vi "start.vi"(8 "error in (no error)":errorcluster, 11 "CQT_DDS in":refnum<class "CQT_DDS.lvclass">) -> (0 "error out":errorcluster, 3 "CQT_DDS out":refnum<class "CQT_DDS.lvclass">)   [LabVIEW 2011, in "CQT_DDS.lvclass"]
uses:
  CQT_DDS.lvclass
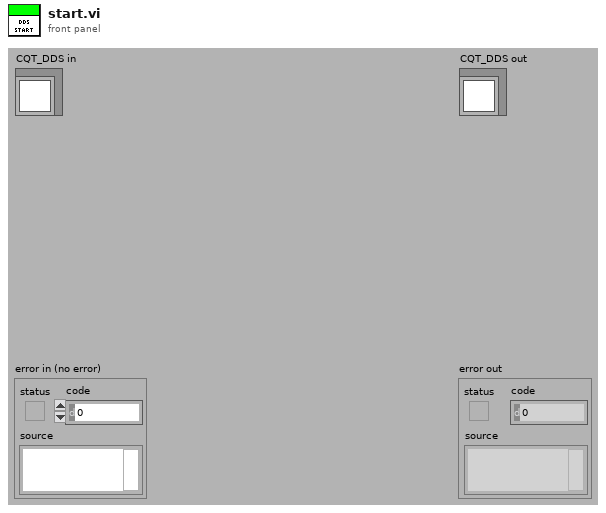
[diagram p1: front panel]
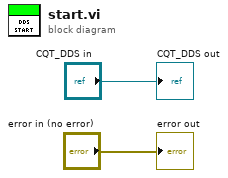
[diagram p0: block diagram]
diagram:
  "error out" <- "error in (no error)"
  "CQT_DDS out" <- "CQT_DDS in"
